vi "Set Server Stop UE.vi"(10 "Server Stop UE":refnum<user-event>, 11 "OOP Server in":refnum<class "OCVTest.lvclass">) -> (3 "OOP Server out":refnum<class "OCVTest.lvclass">)   [LabVIEW 2019, in "OCVTest.lvlib" / "OCVTest.lvclass"]
uses:
  OCVTest.lvclass
  OCVTest.lvclass/OCVTest.ctl
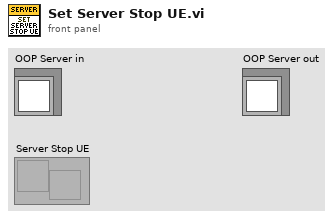
[diagram p1: front panel]
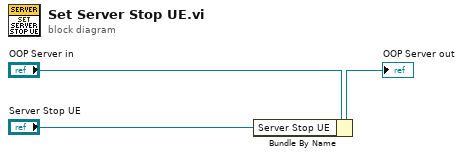
[diagram p0: block diagram]
diagram:
  n1 = Bundle By Name(cluster="OOP Server in", "Server Stop UE"="Server Stop UE") -> (→"OOP Server out":refnum<class "OCVTest.lvclass">)
